vi "Osciloscope setup.vi"(8 "error in (no error)":errorcluster) -> (0 "error out":errorcluster, 3 "Module ID":i32)   [LabVIEW 2020]
doc: "_____\nCreated using DQMH Event Scripter 6.0.0.122."
uses:
  Libraries/Osciloscope/Osciloscope.lvlib
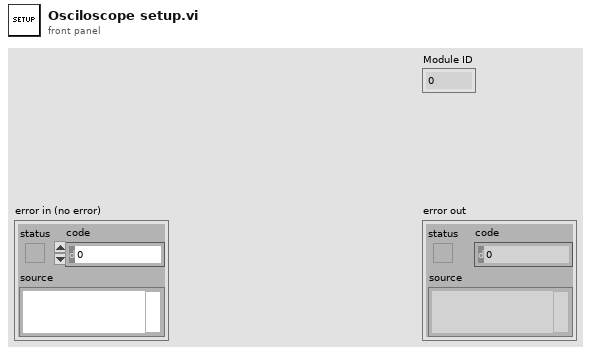
[diagram p1: front panel]
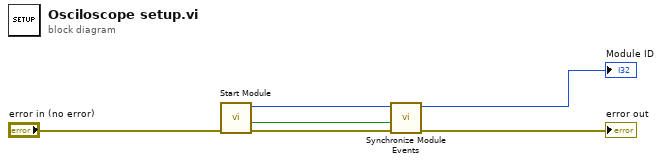
[diagram p0: block diagram]
diagram:
  n1 = call "Start Module.vi"("error in"="error in (no error)") -> ("error out"=w5:errorcluster, "Wait for Event Sync?"=w1:bool, "Module ID"=w2:i32)  [unwired: 7 in, 1 out]
  n2 = call "Synchronize Module Events.vi"("error in"=w5, "Wait for Event Sync?"=w1, "Module ID in"=w2) -> ("error out"=→"error out":errorcluster, "Module ID out"=→"Module ID":i32)  [unwired: 7 in]
